vi "Notify.vi"(8 "error in (no error)":errorcluster, 9 "ErrorOrSuccess":refnum<class "ErrorOrSuccess.lvclass">, 10 "SubscriptionDetailsParent":refnum<class "SubscriptionDetailsParent.lvclass">, 11 "Subscribe JSON in":refnum<class "Subscribe JSON.lvclass">) -> (0 "error out":errorcluster, 3 "Subscribe JSON out":refnum<class "Subscribe JSON.lvclass">)   [LabVIEW 2020, in "wamplv.lvlib" / "Subscribe JSON.lvclass"]
uses:
  Subscribe JSON.lvclass
  Subscribe JSON.lvclass/Subscribe JSON.ctl
  Message loop classes/Subscription details/SubscriptionDetails JSON/SubscriptionDetails JSON.lvclass
  Message loop classes/ErrorOrSuccess JSON/ErrorOrSuccess JSON.lvclass
  Subscribe result (JSON).ctl
  wamplv.lvlib
  Message loop classes/Subscription details/SubscriptionDetailsParent/SubscriptionDetailsParent.lvclass
  Message loop classes/ErrorOrSuccess/ErrorOrSuccess.lvclass
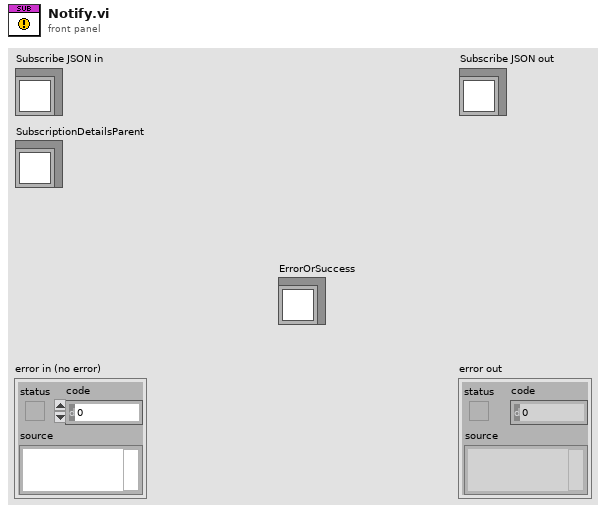
[diagram p1: front panel]
types:
  T1 = typedef "wamplv.lvlib/Subscribe result (JSON).ctl" = cluster{"SubscriptionDetails JSON":refnum<class "SubscriptionDetails JSON.lvclass">, "ErrorOrSuccess JSON":refnum<class "ErrorOrSuccess JSON.lvclass">}
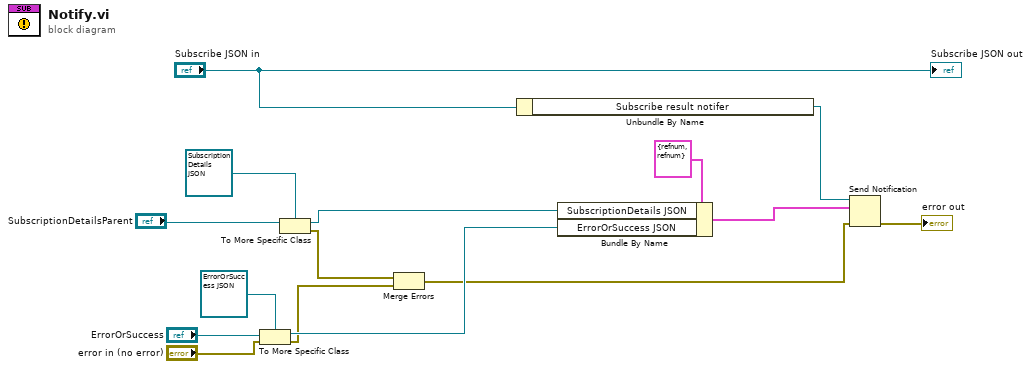
[diagram p0: block diagram]
diagram:
  n1 = To More Specific Class(target class=refnum<class "ErrorOrSuccess JSON.lvclass"> refnum ("wamplv.lvlib:ErrorOrSuccess JSON.lvclass"), reference="ErrorOrSuccess", error in="error in (no error)") -> (specific class reference=w4:refnum<class "ErrorOrSuccess JSON.lvclass">, error out=w2:errorcluster)
  n2 = To More Specific Class(target class=refnum<class "SubscriptionDetails JSON.lvclass"> refnum ("wamplv.lvlib:SubscriptionDetails JSON.lvclass"), reference="SubscriptionDetailsParent") -> (specific class reference=w8:refnum<class "SubscriptionDetails JSON.lvclass">, error out=w3:errorcluster)  [unwired: 1 in]
  n3 = Merge Errors(w3, w2) -> (w1:errorcluster)
  n4 = Unbundle By Name("Subscribe JSON in") -> ("Subscribe result notifer"=w12:refnum<notifier>)
  n5 = Bundle By Name(cluster=T1 {"SubscriptionDetails JSON"=refnum, "ErrorOrSuccess JSON"=refnum} ("Subcsribe Result JSON"), "SubscriptionDetails JSON"=w8, "ErrorOrSuccess JSON"=w4) -> (w9:T1)
  n6 = Send Notification(notification=w9, notifier=w12, error in (no error)=w1) -> (error out=→"error out":errorcluster)  [unwired: 1 out]
  "Subscribe JSON out" <- "Subscribe JSON in"
